vi "CreatePublicEvents.vi"(8 "error in (no error)":errorcluster, 11 "Instrument.Temperhum":refnum<class "Instrument.Temperhum.lvclass">) -> (0 "error out":errorcluster, 3 "Instrument.Temperhum out":refnum<class "Instrument.Temperhum.lvclass">)   [LabVIEW 2019, in "Instrument.Temperhum.lvclass"]
doc: "---------------------------------------------------------------\nJKI State Machine Objects™\nhttp://jki.net/state-machine-objects/\nCopyright (C) 2005-2015, JKI <info@jki.net>\nALL RIGHTS RESERVEDJKI State Machine Objects (SMO) 1.0.0.4\nJKI - JKI\nCopyright (c) 2015, JKI"
uses:
  Instrument.Temperhum.lvclass
  Typedefs/PublicEvents--Instrument.Temperhum.Get PGSQL Info.ctl
  Instrument.Temperhum.lvclass/Instrument.Temperhum.ctl
  <userlib>/LevyLab/Instrument Framework/Instrument Types/VSource/Instrument.VSource.lvclass
panel:
  # "For instructions on how to use the JKI State Machine Objects, examples and video tutorials, visit:\nhttp://jki.net/state-machine-objects/\n\nJKI State Machine Objects™\nhttp://jki.net/state-machine-objects/\nCopyright (C) 2005-2015, JKI <info@jki.net>\nALL RIGHTS RESERVED"
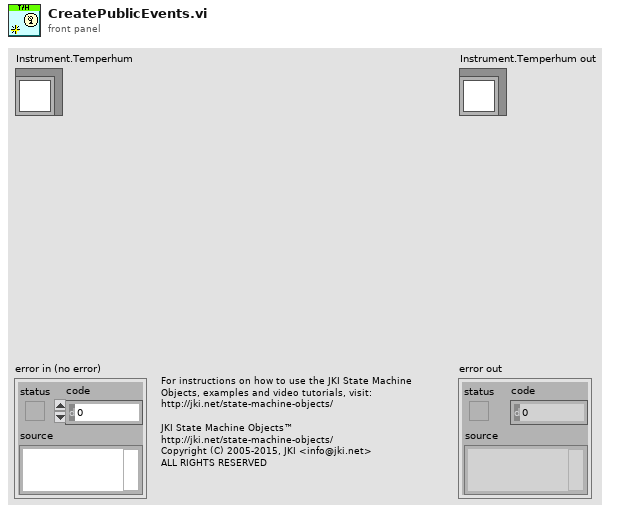
[diagram p1: front panel]
types:
  T1 = typedef "Instrument.Temperhum.lvclass/PublicEvents--Instrument.Temperhum.Get PGSQL Info.ctl" = string
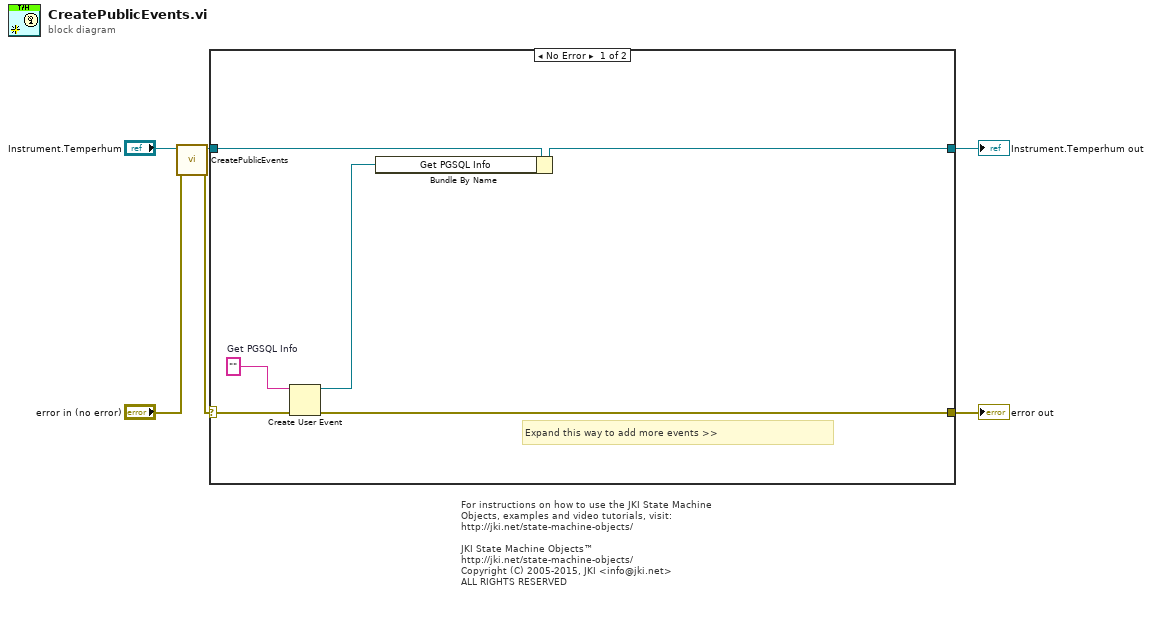
[diagram p0: block diagram]
diagram:
  # "For instructions on how to use the JKI State Machine Objects, examples and video tutorials, visit:\nhttp://jki.net/state-machine-objects/\n\nJKI State Machine Objects™\nhttp://jki.net/state-machine-objects/\nCopyright (C) 2005-2015, JKI <info@jki.net>\nALL RIGHTS RESERVED"
  n1 = call-parent "CreatePublicEvents.vi"("error in (no error)"="error in (no error)", "Instrument"="Instrument.Temperhum") -> ("error out"=w1:errorcluster, "Instrument out"=w3:refnum<class "Instrument.Temperhum.lvclass">)  [unwired: 8 in]
  n2 = case shown="No Error" w1 {
    selector: w1 -> [w11 w14]
    tunnel: [w9 w14] -> w5
    tunnel: [w10 w13] -> w6
    tunnel: w3 -> [w12 w13]
    frame No Error {
      w7 = T1 ""  # Get PGSQL Info
      # "Expand this way to add more events >>"
      n3 = Create User Event(user event datatype=w7, error in=w11) -> (user event=w8:refnum<user-event>, error out=w9:errorcluster)
      n4 = Bundle By Name(cluster=w12, "Get PGSQL Info"=w8) -> (w10:refnum<class "Instrument.Temperhum.lvclass">)
    }
    frame Error {
    }
  }
  "error out" <- w5
  "Instrument.Temperhum out" <- w6
